vi "oax_gsShaft Center Line.vi"() -> ()   [LabVIEW 2017]
doc: "This example shows how to display shaft certerline plot with the logged vibration and tachometer signals."
uses:
  <vilib>/addons/Sound and Vibration/Order Analysis/Tach Process/SoundVib_TachProcess.lvlib
  <vilib>/addons/Sound and Vibration/svt_Calibration/SoundVib_Calibration.lvlib
  <vilib>/addons/Sound and Vibration/Order Analysis/Utility/SubVIs/oa_Buffer Settings.ctl
  <vilib>/addons/Sound and Vibration/Order Analysis/Utility/SoundVib_OAUtility.lvlib
  <vilib>/addons/Sound and Vibration/Order Analysis/Resample Order Tracking/SoundVib_OrderTracking.lvlib
  <vilib>/addons/Sound and Vibration/Order Analysis/Referece Data Processing/SoundVib_RefDataProcess.lvlib
  <vilib>/addons/Sound and Vibration/Order Analysis/Data Presentation/SoundVib_MCMDisplay.lvlib
  <vilib>/addons/Sound and Vibration/Order Analysis/Data Presentation/SubVIs/OAT MCM Channel Property.ctl
  <vilib>/addons/_XControls/Shaft Centerline/SVX SC Line.xctl
  <vilib>/addons/Sound and Vibration/Order Analysis/Tach Process/SubVIs/digital tach info.ctl
panel:
  in  "clearance boundary settings":T1={"boundary"={"x axis"=0.01, "y axis"=0.01}, "start point"=enum."bottom"}
  in  "Select Data":i32(listbox)
  in  "output cluster":T3
  out "gap unit":string="mm"
  in  "plot label selection":u16(ring)=2 items=["Time", "Revolution", "RPM"]
  out "Y- axis":dbl
  out "X- axis":dbl
  out "Speed Profile":cluster{"time [s]":dbl[], "speed [rpm]":dbl[]}(graph)
  out "Shaft Centerline Plot":T4(xcontrol)=[{"probe x"=[], "probe y"=[], "reference"=[], "attribute"=variant("NI_OAT_Angle_X"=variant(u16 0), "NI_OAT_Angle_Y"=variant(u16 90), "NI_OAT_Direction"=variant(u16 0), "NI_OAT_Pair"=variant(string "0"), "NI_OAT_X_Axis"=variant(string "RPM"))}]
  in  "STOP":bool
  # "Reference Voltage [V]"
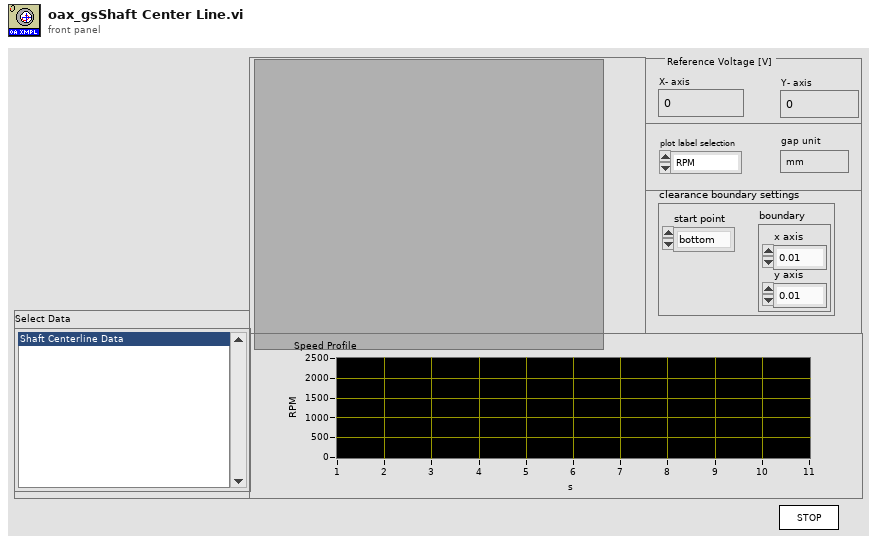
[diagram p1: front panel]
types:
  T1 = cluster{"boundary":cluster{"x axis":dbl, "y axis":dbl}, "start point":enum16{"center", "top", "bottom"}}
  T2 = typedef "SoundVib_TachProcess.lvlib/digital tach info.ctl" = cluster{"tacho counts":i64[], "counter timebase [Hz]":dbl, "counter task type":enum16{"period measurement", "event counting"}, "counter digit (32)":i32}
  T3 = cluster{"digital tacho info":T2, "waveform data":waveform(dbl)[]}
  T4 = cluster{"probe x":dbl[], "probe y":dbl[], "reference":dbl[], "attribute":variant}[]
  T5 = typedef "OAT MCM Channel Property.ctl" = cluster{"direction":u16, "probe angle [deg]":u16, "pair":u16}
  T6 = enum16{"Rectangular (none)", "Hanning", "Low side lobe"}
  T7 = typedef "SoundVib_OAUtility.lvlib/oa_Buffer Settings.ctl" = cluster{"buffer size":dbl, "buffer unit":enum16{"s", "revolution", "# of samples"}}
  T8 = typedef "svc_Channel Info.ctl" = cluster{"sensor sensitivity":dbl, "engineering units":T9, "dB reference":dbl, "custom label":string, "weighting filter":T10, "pregain":dbl}
  T9 = typedef "svc_Engineering Units Text Ring.ctl" = u16
  T10 = typedef "svc_Weighting Filter Text Ring.ctl" = u16
  T11 = typedef "SoundVib_TachProcess.lvlib/speed profile.ctl" = cluster{"time [s]":dbl[], "speed [RPM]":dbl[]}
  T12 = typedef "OAT Position Info.ctl" = cluster{"positions [s]":dbl[], "samples/rev":dbl}
  T13 = typedef "svc_Resampled Channel Info.ctl" = cluster{"channel name":string, "description":string, " channel info":T8}
  T14 = cluster{"time/rev/rpm":dbl[], "DC gap value":dbl[]}[]
  T15 = cluster{"x unit":string, "DC gap unit out":string}[]
  T16 = cluster{"x unit":string, "DC gap unit out":string}
  T17 = cluster{"boundary":cluster{"x axis":dbl, "y axis":dbl}, "start point":enum16{"center", "top", "bottom"}}[]
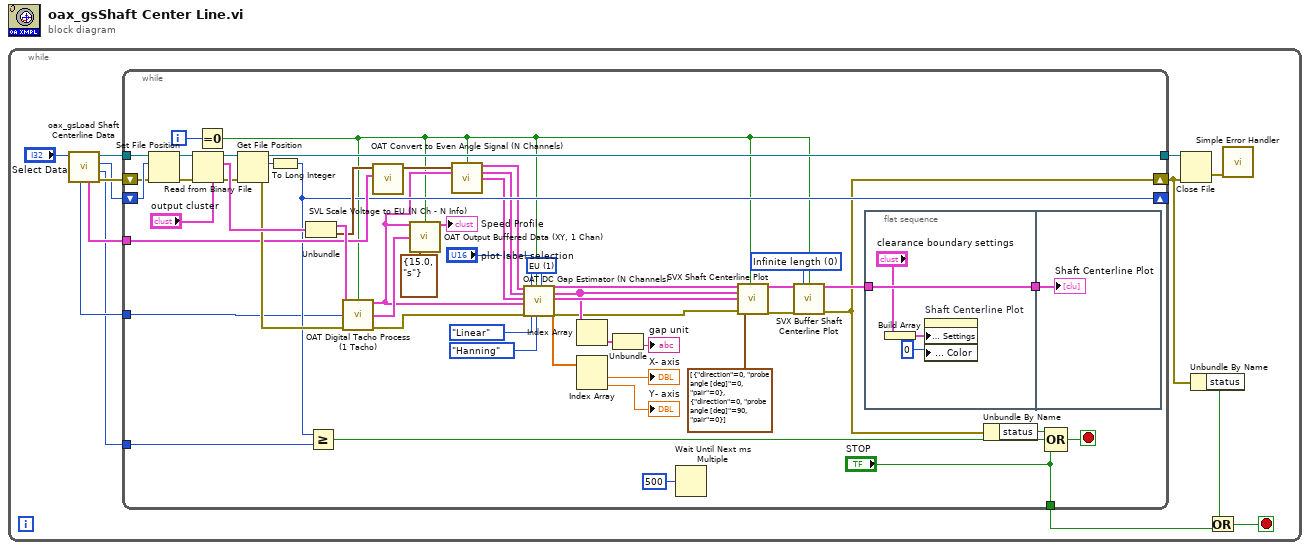
[diagram p0: block diagram]
diagram:
  n1 = while {
    stop <- w3 stop-if-true
    n2 = call <vilib>:"oax_gsLoad Shaft Centerline Data.vi"("data type"="Select Data") -> ("error out"=w11:errorcluster, "end position"=w6:i32, "current position"=w10:i32, "refnum"=w12:refnum<file>, "channel info"=w9:T8[], "pulse / rev"=w8:i32)  [unwired: 4 in, 1 out]
    n3 = while {
      tunnel: w12 -> [w67]
      shift-right: [w47] -> _
      shift-left: w10 -> [w66]
      tunnel: [w64] -> w13
      shift-right: [w16] -> w5
      shift-left: w11 -> [w61]
      tunnel: w9 -> [w48]
      tunnel: w8 -> [w41]
      tunnel: w6 -> [w46]
      tunnel: ["STOP"] -> w2
      i -> [w63]
      stop <- w39 stop-if-true
      w14 = u16 0 items=["Infinite length", "Last block data", "Custom"] ("buffer mode")
      w58 = u16 1 items=["V", "EU"] ("DC gap unit")
      n4 = Set File Position(offset (in bytes) (0)=w66, refnum=w67, error in=w61) -> (refnum out=w32:refnum<file>, error out=w31:errorcluster)  [unwired: 1 in]
      n5 = Read from Binary File(5:"output cluster", 8:w31, 11:w32) -> (0:w29:errorcluster, 2:w62:T3, 3:w30:refnum<file>)  [unwired: 3 in, 1 out]
      n6 = Equal To 0?(x=w63) -> (x = 0?=w15:bool)
      n7 = Get File Position(4:w29, 7:w30) -> (0:w52:errorcluster, 2:w28:i64, 3:w64:refnum<file>)
      n8 = To Long Integer(number=w28) -> (32bit integer=w47:i32)
      n9 = Unbundle(w62) -> ("digital tacho info"=w60:T2, "waveform data"=w49:waveform(dbl)[])
      n10 = Greater Or Equal?(x=w47, y=w46) -> (x >= y?=w44:bool)
      n11 = call <vilib>:"OAT Digital Tacho Process (1 Tacho).vi"("digital tacho info"=w60, "reset? (F)"=w15, "pulse/revolution (1)"=w41, "error in (no error)"=w52) -> ("speed profile"=w27:T11, "speed position info"=w37:T12, "error out"=w59:errorcluster)  [unwired: 8 in, 1 out]
      n12 = call <vilib>:"SVL Scale Voltage to EU (N Ch - N Info).vi"("channel info"=w48, "signals [V]"=w49) -> ("scaled signals [EU]"=w35:waveform(dbl)[])  [unwired: 7 in, 2 out]
      n13 = call <vilib>:"OAT Output Buffered Data (XY, 1 Chan).vi"("XY signal"=w27, "reset? (F)"=w15, "position info"=w37, "buffer settings"=T7 {"buffer size"=15.0, "buffer unit"=enum."s"}) -> ("buffered XY signal"=→"Speed Profile":cluster{"X":dbl[], "Y":dbl[]})  [unwired: 9 in, 2 out]
      n14 = call <vilib>:"OAT Convert to Even Angle Signal (N Channels).vi"("scaled signals [EU]"=w35, "reset? (F)"=w15, "speed profile"=w27) -> ("even-angle signals"=w34:cluster{"r0":dbl, "dr":dbl, "Y":dbl[]}[], "even-angle channel info"=w33:T13[], "even-angle position info"=w36:T12)  [unwired: 8 in, 2 out]
      n15 = call <vilib>:"OAT DC Gap Estimator (N Channels).vi"("even-angle signals"=w34, "even-angle channel info"=w33, "even-angle position info"=w36, "speed profile"=w27, "error in (no error)"=w59, "x-axis selection"="plot label selection", "averaging type"=enum16{"Linear", "Exponential"}."Linear", "reset? (F)"=w15, "window"=T6."Hanning", "DC gap unit"=w58) -> ("DC gaps"=w21:T14, "unit labels"=w23:T15, "gap position info"=w24:T12, "actual gap ref [V]"=w55:dbl[], "error out"=w20:errorcluster)  [unwired: 5 in]
      n16 = Index Array(array=w23) -> (element=w51:T16)  [unwired: 1 in]
      n17 = Index Array(array=w55) -> (element #1=→"X- axis":dbl, element #2=→"Y- axis":dbl)  [unwired: 2 in]
      n18 = Unbundle(w51) -> ("DC gap unit out"=→"gap unit":string)  [unwired: 1 out]
      n19 = Wait Until Next ms Multiple(millisecond multiple=u32 500) -> ()  [unwired: 1 out]
      n20 = call <vilib>:"SVX Shaft Centerline Plot.vi"("DC gaps"=w21, "unit labels"=w23, "gap position info"=w24, "error in (no error)"=w20, "channel properties"=T5[] [{"direction"=0, "probe angle [deg]"=0, "pair"=0}, {"direction"=0, "probe angle [deg]"=90, "pair"=0}], "reset? (F)"=w15) -> ("shaft centerline"=w19:T4, "error out"=w18:errorcluster)  [unwired: 12 in]
      n21 = call <vilib>:"SVX Buffer Shaft Centerline Plot.vi"("shaft centerline in"=w19, "buffer mode"=w14, "reset? (F)"=w15, "error in (no error)"=w18) -> ("shaft centerline out"=w17:T4, "error out"=w16:errorcluster)  [unwired: 10 in]
      n22 = flat-sequence {
        tunnel: w17 -> [w71]
        tunnel: [w71] -> w22
        tunnel: w22 -> [w72]
        frame #0 {
          n23 = Build Array("clearance boundary settings") -> (w70:T17)
          n24 = property on="Shaft Centerline Plot"("Clearance Boundary: Settings"=w70, "Clearance Boundary: Color"=u32 0) -> ()  [unwired: 2 in, 2 out]
        }
        frame #1 {
          "Shaft Centerline Plot" <- w72
        }
      }
      n25 = Unbundle By Name(w16) -> ("status"=w45:bool)
      n26 = Compound Arithmetic op=OR(w45, w44, "STOP") -> (w39:bool)
    }
    n27 = Close File(refnum=w13, error in=w5) -> (error out=w7:errorcluster)  [unwired: 1 out]
    n28 = Unbundle By Name(w5) -> ("status"=w4:bool)
    n29 = Or(x=w4, y=w2) -> (x .or. y?=w3:bool)
    n30 = call <vilib>:"Simple Error Handler.vi"("error in (no error)"=w7) -> ()  [unwired: 4 in, 5 out]
  }
